vi "main1.vi"() -> ()   [LabVIEW 2019]
panel:
  out "Array 2":string[](array[string])
  in  "stop":bool
  out "B7 chiffre":string
  out "B8 chiffre":string
  out "B9 chiffre":string
  out "B6 chiffre":string
  out "B4 chiffre":string
  out "B3 chiffre":string
  out "B2 chiffre":string
  out "B1 chiffre":string
  out "W4 chiffre":string
  out "W6 chiffre":string
  out "W1 chiffre":string
  out "W2 chiffre":string
  out "W3 chiffre":string
  out "R3 chiffre":string
  out "R6 chiffre":string
  out "R8 chiffre":string
  out "R9 chiffre":string
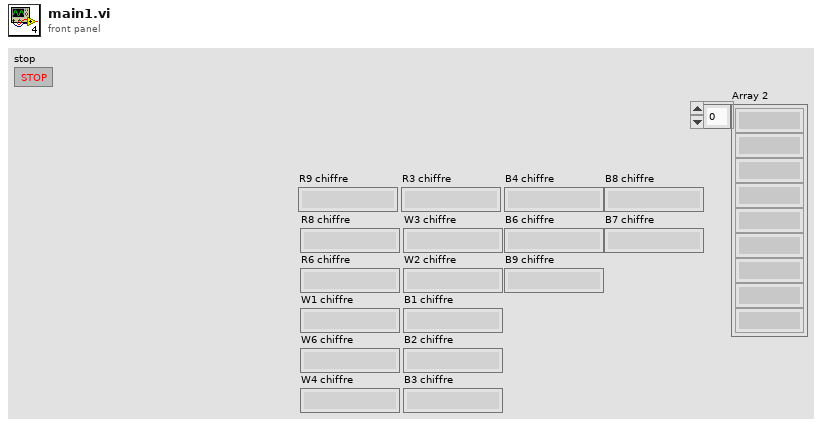
[diagram p1: front panel]
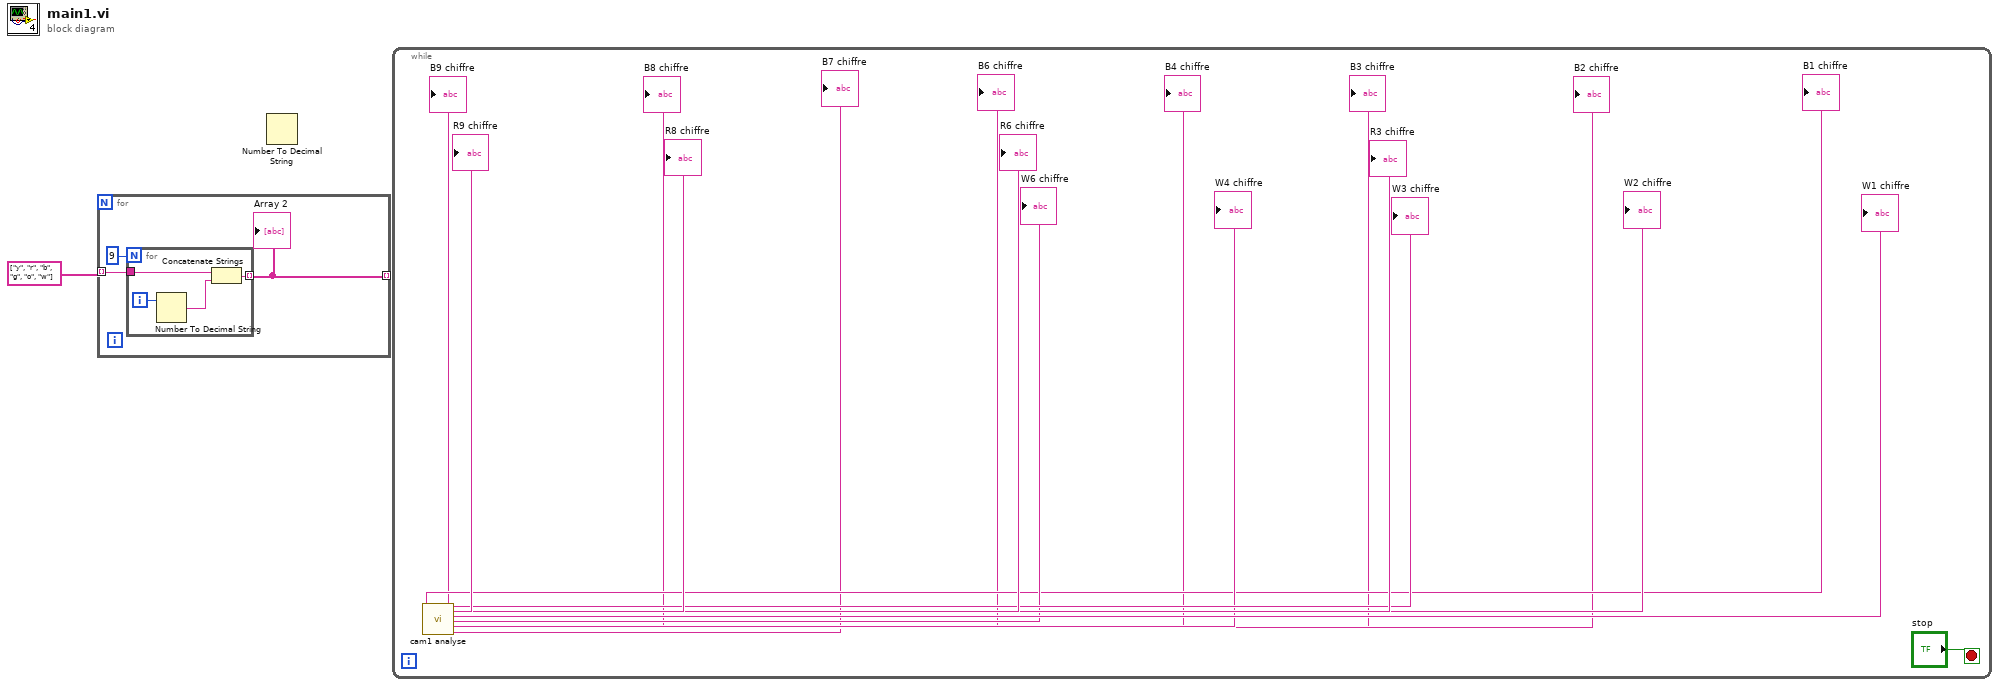
[diagram p0: block diagram]
diagram:
  n1 = for {
    tunnel: string[] ["y", "r", "b", "g", "o", "w"] -> [w4] mode=indexing
    tunnel: [w2] -> _ mode=indexing
    n2 = for {
      N: 9 -> [_]
      tunnel: w4 -> [w7]
      tunnel: [w5] -> w2 mode=indexing
      i -> [w8]
      n3 = Number To Decimal String(number=w8) -> (decimal integer string=w6:string)  [unwired: 1 in]
      n4 = Concatenate Strings(w7, w6) -> (w5:string)
    }
    "Array 2" <- w2
  }
  n5 = Number To Decimal String() -> ()  [unwired: 2 in, 1 out]
  n6 = while {
    stop <- "stop" stop-if-true
    n7 = call "cam1 analyse.vi"() -> ("W3 chiffre"=→"W3 chiffre":string, "W2 chiffre"=→"W2 chiffre":string, "W1 chiffre"=→"W1 chiffre":string, "W6 chiffre"=→"W6 chiffre":string, "W4 chiffre"=→"W4 chiffre":string, "B1 chiffre"=→"B1 chiffre":string, "R3 chiffre"=→"R3 chiffre":string, "B2 chiffre"=→"B2 chiffre":string, "R6 chiffre"=→"R6 chiffre":string, "B3 chiffre"=→"B3 chiffre":string, "R8 chiffre"=→"R8 chiffre":string, "B4 chiffre"=→"B4 chiffre":string, "R9 chiffre"=→"R9 chiffre":string, "B6 chiffre"=→"B6 chiffre":string, "B9 chiffre"=→"B9 chiffre":string, "B8 chiffre"=→"B8 chiffre":string, "B7 chiffre"=→"B7 chiffre":string)  [unwired: 3 in]
  }
